vi "ConfigInstr.vi"(6 "InstrumentName":string, 7 "VisaRessIn":refnum<visa-resource-name>, 8 "error in (no error)":errorcluster caption="entrée d'erreur (pas d'erreur)", 9 "FirstClassInst":bool, 10 "Function":string, 11 "GenData In":refnum<class "YokoGS200.lvclass"> caption="DNL_LabVIEW Object in") -> (0 "error out":errorcluster caption="sortie d'erreur", 3 "GenData Out":refnum<class "YokoGS200.lvclass"> caption="DNL_LabVIEW Object out")   [LabVIEW 2019, in "YokoGS200.lvclass"]
uses:
  YokoGS200.lvclass
  C:/Programmes Labview/LabScanV1A/DevicesClass/BaseDevice/BaseDevice.lvclass
  YokoGS200_Func.ctl
  YokoGS200.lvclass/YokoGS200.ctl
  BaseDevice/BaseDevice.lvclass/BaseDevice.ctl
  BaseDevice/Accessor/SetShowInstrNm.vi
  BaseDevice/Accessor/SetInstrParam.vi
panel:
  in  "Class_Func":T1
  out "VisaRessOut":refnum<visa-resource-name>
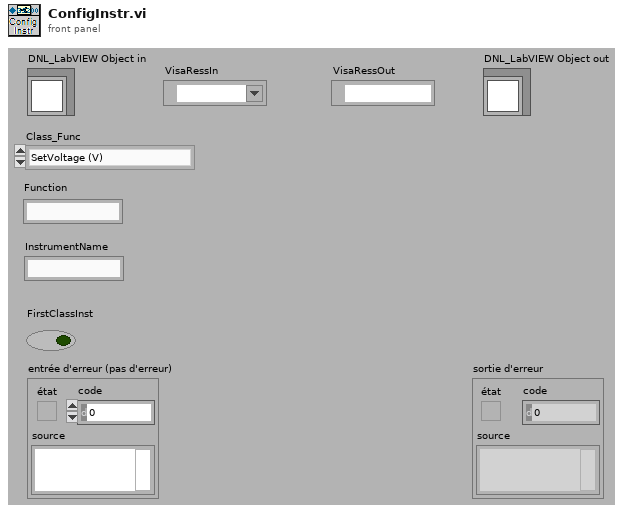
[diagram p1: front panel]
types:
  T1 = typedef "YokoGS200.lvclass/YokoGS200_Func.ctl" = enum16{"SetVoltage (V)", "SetCurrent (A)"}
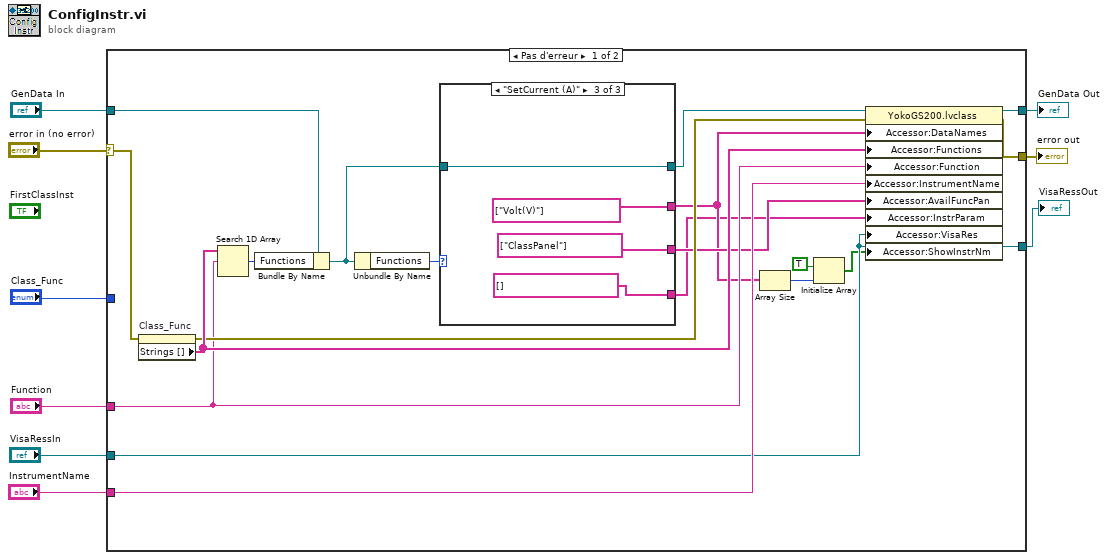
[diagram p0: block diagram]
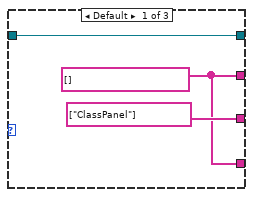
[diagram p2: hidden frame]
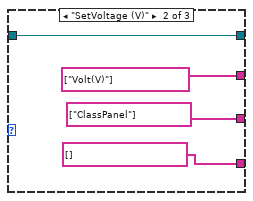
[diagram p3: hidden frame]
diagram:
  n1 = case shown="Pas d'erreur" "error in (no error)" {
    selector: "error in (no error)" -> [w22 w41]
    tunnel: [w28 w41] -> w8
    tunnel: "GenData In" -> [w23 w40]
    tunnel: [w27 w40] -> w6
    tunnel: "Class_Func" -> [_ _]
    tunnel: "Function" -> [w18 _]
    tunnel: "InstrumentName" -> [w17 _]
    tunnel: "VisaRessIn" -> [w15 _]
    tunnel: [w15 _] -> w1
    frame No Error {
      n2 = property on="Class_Func" class="Énum (strict)"(error in=w22) -> (error out=w21:errorcluster, "Strings []"=w25:string[])  [unwired: 1 in, 1 out]
      n3 = Search 1D Array(1D array=w25, element=w18) -> (index of element=w24:i32)  [unwired: 1 in]
      n4 = Bundle By Name(cluster=w23, "Functions"=w24) -> (w20:refnum<class "YokoGS200.lvclass">)
      n5 = Unbundle By Name(w20) -> ("Functions"=w26:T1)
      n6 = case shown="\"SetCurrent (A)\"" w26 {
        tunnel: [w29 string[] ["Volt(V)"] string[] ["Volt(V)"]] -> w12
        tunnel: w20 -> [w31 w35 w39]
        tunnel: [w31 w35 w39] -> w19
        tunnel: [string[] ["ClassPanel"] string[] ["ClassPanel"] string[] ["ClassPanel"]] -> w16
        tunnel: [w29 string[] [] string[] []] -> w10
        frame Default {
          w29 = string[] []
        }
        frame "SetVoltage (V)" {
        }
        frame "SetCurrent (A)" {
        }
      }
      n7 = Array Size(array=w12) -> (size(s)=w14:i32)
      n8 = Initialize Array(TRUE, w14) -> (w11:bool[])
      n9 = property class="YokoGS200.lvclass"(reference=w19, error in=w21, "Accessor:DataNames"=w12, "Accessor:Functions"=w25, "Accessor:Function"=w18, "Accessor:InstrumentName"=w17, "Accessor:AvailFuncPan"=w16, "Accessor:InstrParam"=w10, "Accessor:VisaRes"=w15, "Accessor:ShowInstrNm"=w11) -> (reference out=w27:refnum<class "YokoGS200.lvclass">, error out=w28:errorcluster)
    }
    frame Error {
    }
  }
  "error out" <- w8
  "GenData Out" <- w6
  "VisaRessOut" <- w1
